vi "Wait.vi"(8 "error in (no error)":errorcluster, 10 "Wait (1mS)":u32=1, 11 "VISA resource name":refnum<visa-resource-name>) -> (0 "error out":errorcluster, 3 "VISA resource name out":refnum<visa-resource-name>)   [LabVIEW 2012, in "TDK-Lambda Z.lvlib"]
doc: "Waits a number of milliseconds. Used for allowing instrument to settle after changing the output. If \"Delay\" input not wired, it will wait 1 mSec."
uses:
  TDK-Lambda Z.lvlib
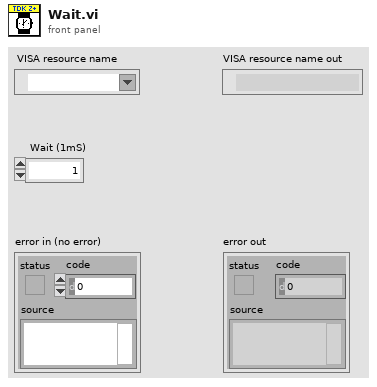
[diagram p1: front panel]
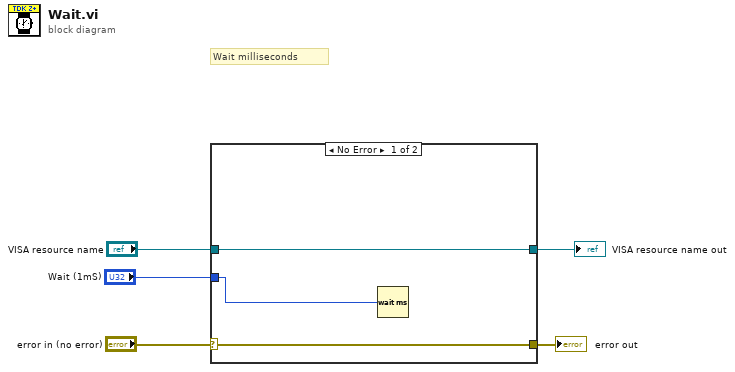
[diagram p0: block diagram]
diagram:
  # "Wait milliseconds"
  n1 = case shown="No Error" "error in (no error)" {
    selector: "error in (no error)" -> [w8 w9]
    tunnel: [w8 w9] -> w2
    tunnel: "VISA resource name" -> [w7 w10]
    tunnel: [w7 w10] -> w3
    tunnel: "Wait (1mS)" -> [w6 _]
    frame No Error {
      n2 = Wait (ms)(milliseconds to wait=w6) -> ()  [unwired: 1 out]
    }
    frame Error {
      # "If Error Exists,  Do Not Wait"
    }
  }
  "error out" <- w2
  "VISA resource name out" <- w3
